vi "Reset.vi"(8 "error in (no error)":errorcluster, 10 "Message in":refnum<class "ResetMessage.lvclass">, 11 "Galvo in":refnum<class "InVivo_ImagingModeSPIM.lvclass">) -> (0 "error out":errorcluster, 3 "Galvo out":refnum<class "InVivo_ImagingModeSPIM.lvclass">)   [LabVIEW 2012, in "InVivo_ImagingModeSPIM.lvclass"]
doc: "The reset method processes the command 'reset'. \n\nResets the internal state of the component (without performing a full initialisation). This could be resetting hardware, or private data to default values."
uses:
  InVivo_ImagingModeSPIM.lvclass
  <vilib>/Distrio/Murmex/ResetMessage/ResetMessage.lvclass
  <vilib>/Distrio/Murmex/Murmex/Murmex.lvclass
  <vilib>/Distrio/Murmex/StopMessage/StopMessage.lvclass
  <vilib>/Distrio/Murmex/StartMessage/StartMessage.lvclass
panel:
  # "This method is called when the RESET\ntrigger is sent. \n\nOverride this method when your component needs to\nrespond to this trigger. \n\nCall parent for proper implementation"
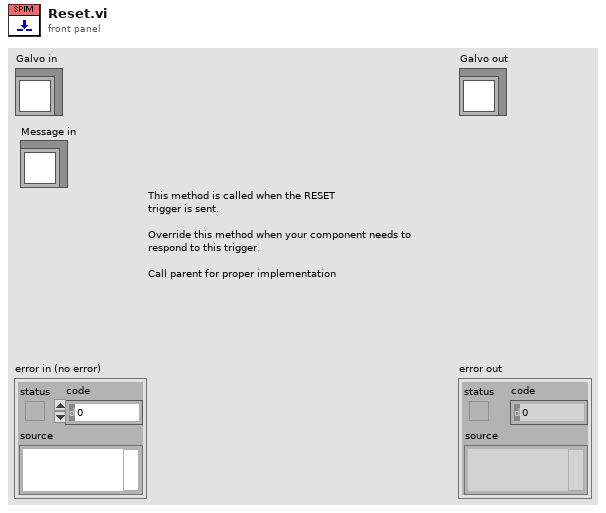
[diagram p1: front panel]
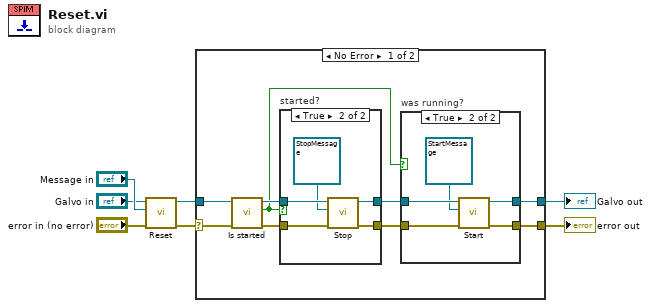
[diagram p0: block diagram]
diagram:
  n1 = call-parent "Reset.vi"("error in (no error)"="error in (no error)", "Message in"="Message in", "Murmex in"="Galvo in") -> ("error out"=w1:errorcluster, "Murmex out"=w3:refnum<class "InVivo_ImagingModeSPIM.lvclass">)  [unwired: 7 in]
  n2 = case shown="No Error" w1 {
    selector: w1 -> [w12 w32]
    tunnel: [w16 w32] -> w4
    tunnel: w3 -> [w14 w31]
    tunnel: [w15 w31] -> w2
    frame No Error {
      n3 = call <vilib>:"Is started.vi"("error in (no error)"=w12, "Murmex in"=w14) -> ("error out"=w11:errorcluster, "started?"=w10:bool, "Murmex out"=w13:refnum<class "InVivo_ImagingModeSPIM.lvclass">)  [unwired: 7 in]
      n4 = case "started?" shown="True" w10 {
        tunnel: [w24 w30] -> w9
        tunnel: [w25 w29] -> w8
        tunnel: w13 -> [w25 w28]
        tunnel: w11 -> [w24 w27]
        frame False {
        }
        frame True {
          n5 = call-dynamic "Stop.vi"("error in (no error)"=w27, "Message in"=refnum<class "StopMessage.lvclass"> refnum ("Murmex.lvlib:StopMessage"), "Galvo in"=w28) -> ("error out"=w30:errorcluster, "Galvo out"=w29:refnum<class "InVivo_ImagingModeSPIM.lvclass">)  [unwired: 7 in]
        }
      }
      n6 = case "was running?" shown="True" w10 {
        tunnel: [w17 w23] -> w16
        tunnel: [w18 w22] -> w15
        tunnel: w8 -> [w18 w21]
        tunnel: w9 -> [w17 w20]
        frame False {
        }
        frame True {
          n7 = call-dynamic "Start.vi"("error in (no error)"=w20, "Message in"=refnum<class "StartMessage.lvclass"> refnum ("Murmex.lvlib:StartMessage"), "Galvo in"=w21) -> ("error out"=w23:errorcluster, "Galvo out"=w22:refnum<class "InVivo_ImagingModeSPIM.lvclass">)  [unwired: 7 in]
        }
      }
    }
    frame Error {
    }
  }
  "error out" <- w4
  "Galvo out" <- w2
